vi "Joystick-Manual-Client.vi"() -> ()   [LabVIEW 2012]
doc: "Use this VI with the UDP Sender VI. Run this VI first.\n\nThe UDP protocol differs from TCP in that there is no error-checking with the packets of information that are sent, and thus no guarantee whatsoever that an intended recipient will actually receive a given piece of data.\n\nUDP does offer the ability to \"broadcast\" data across a network--simply specify an IP Address of all ones (255.255.255.255) to attempt to broadcast information network-wide. Keep in mind that routers and other network hardware will generally refuse to forward the broadcast beyond certain points, so the extent of the broadcast will in practice be limited."
uses:
  <vilib>/Utility/error.llb/DialogType.ctl
  <vilib>/DAQmx/create/channels.llb/DAQmx Create Channel (DO-Digital Output).vi
panel:
  out "Float":bool
  out "rot-":bool
  out "rot+":bool
  out "y-":bool
  out "y+":bool
  out "x-":bool
  out "x+":bool
  in  "Port":u16=61557
  in  "stop":bool
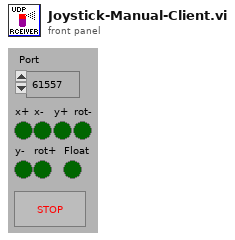
[diagram p1: front panel]
types:
  T1 = typedef "DialogType.ctl" = u16
  T2 = cluster{"x+":bool, "x-":bool, "y+":bool, "y-":bool, "rot+":bool, "rot-":bool, "Float":bool}
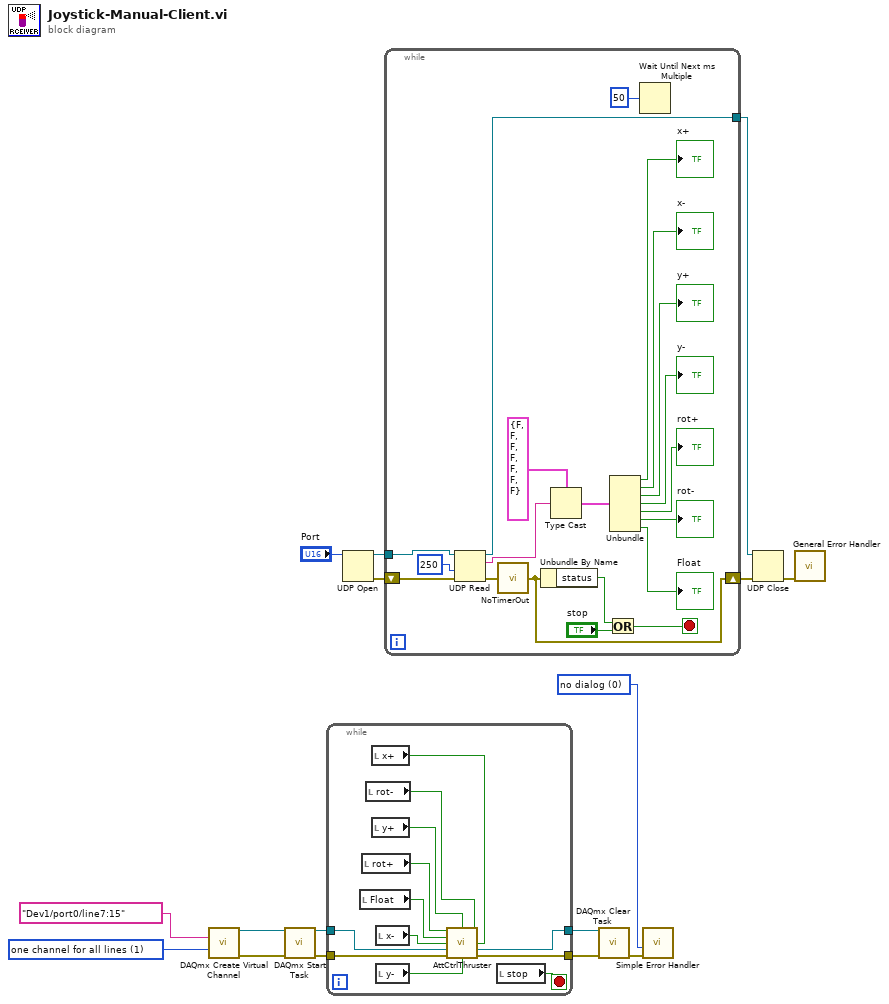
[diagram p0: block diagram]
diagram:
  w4 = T1 0 items=["no dialog", "OK message", "continue or stop message", "OK message + warnings", "continue/stop + warnings"] ("type of dialog (OK msg:1)")
  w9 = 1 items=["one channel for each line", "one channel for all lines"] ("line grouping")
  n1 = call-poly <vilib>:"DAQmx Create Virtual Channel.vi"("lines"=tag "Dev1/port0/line7:15" ("Lines"), "line grouping"=w9) -> ("task out"=w7:refnum<k21>, "error out"=w8:errorcluster)  [unwired: 12 in]
  n2 = call <vilib>:"DAQmx Start Task.vi"("task/channels in"=w7, "error in"=w8) -> ("task out"=w6:refnum<k21>, "error out"=w5:errorcluster)  [unwired: 12 in]
  n3 = while {
    tunnel: w6 -> [w20]
    tunnel: w5 -> [w19]
    tunnel: [w18] -> w2
    tunnel: [w17] -> w1
    stop <- w28 stop-if-true
    n4 = local read "Float"() -> (w27:bool)
    n5 = local read "rot+"() -> (w22:bool)
    n6 = local read "rot-"() -> (w21:bool)
    n7 = local read "x+"() -> (w26:bool)
    n8 = local read "y+"() -> (w24:bool)
    n9 = local read "x-"() -> (w25:bool)
    n10 = local read "y-"() -> (w23:bool)
    n11 = call "AttCtrlThruster.vi"("ctclk"=w22, "Up"=w24, "clkwis"=w21, "Float"=w27, "Left"=w25, "Right"=w26, "task in"=w20, "error in"=w19, "Down"=w23) -> ("task out"=w18:refnum<k21>, "error out"=w17:errorcluster)  [unwired: 5 in]
    n12 = local read "stop"() -> (w28:bool)
  }
  n13 = UDP Open(11:"Port") -> (port=w14:refnum<k16>, 0:w15:errorcluster)  [unwired: 4 in, 1 out]
  n14 = while {
    tunnel: [w48] -> w13
    tunnel: w14 -> [w40]
    shift-left: w15 -> [w39]
    shift-right: [w43] -> w12
    stop <- w46 stop-if-true
    n15 = UDP Read(connection ID=w40, timeout ms (25000)=250, 8:w39) -> (data out=w38:string, error out=w44:errorcluster, 3:w48:refnum<k16>)  [unwired: 1 in, 2 out]
    n16 = call "NoTimerOut.vi"("error in (no error)"=w44) -> ("error out"=w43:errorcluster)
    n17 = Unbundle By Name(w43) -> ("status"=w45:bool)
    n18 = Type Cast(type=T2 {"x+"=FALSE, "x-"=FALSE, "y+"=FALSE, "y-"=FALSE, "rot+"=FALSE, "rot-"=FALSE, "Float"=FALSE} ("output cluster"), x=w38) -> (*(type *) &x=w36:T2)
    n19 = Or(x=w45, y="stop") -> (x .or. y?=w46:bool)
    n20 = Unbundle(w36) -> ("x+"=→"x+":bool, "x-"=→"x-":bool, "y+"=→"y+":bool, "y-"=→"y-":bool, "rot+"=→"rot+":bool, "rot-"=→"rot-":bool, "Float"=→"Float":bool)
    n21 = Wait Until Next ms Multiple(millisecond multiple=u32 50) -> ()  [unwired: 1 out]
  }
  n22 = call <vilib>:"DAQmx Clear Task.vi"("task in"=w2, "error in"=w1) -> ("error out"=w3:errorcluster)  [unwired: 13 in]
  n23 = call <vilib>:"Simple Error Handler.vi"("type of dialog (OK msg:1)"=w4, "error in (no error)"=w3) -> ()  [unwired: 3 in, 5 out]
  n24 = UDP Close(connection ID=w13, 8:w12) -> (error out=w11:errorcluster)  [unwired: 1 out]
  n25 = call <vilib>:"General Error Handler.vi"("error in (no error)"=w11) -> ()  [unwired: 10 in, 5 out]
